vi "Test Cyclic instructions.vi"() -> ()   [LabVIEW 2018]
panel:
  out "Boolean array":bool[](array[boolean])
  out "appended array":string[](array[string])
  in  "String":string="30000"
  in  "cyclic parameter":string
  in  "WPROT positions":cluster{"pos_name":string, "pos_value":dbl}[](array[cluster])=[{"pos_name"="OFFSET", "pos_value"=900.0}, {"pos_name"="WP1", "pos_value"=0.0}, {"pos_name"="WP2", "pos_value"=1875.0}, {"pos_name"="WP3", "pos_value"=3750.0}, {"pos_name"="WP4", "pos_value"=5625.0}, {"pos_name"="WP5", "pos_value"=7500.0}, {"pos_name"="WP6", "pos_value"=9375.0}, {"pos_name"="WP7", "pos_value"=11250.0}, {"pos_name"="WP8", "pos_value"=13125.0}, {"pos_name"="WP9", "pos_value"=15000.0}, {"pos_name"="WP10", "pos_value"=16875.0}, {"pos_name"="WP11", "pos_value"=18750.0}, {"pos_name"="WP12", "pos_value"=20625.0}, {"pos_name"="WP13", "pos_value"=22500.0}, {"pos_name"="WP14", "pos_value"=24375.0}, {"pos_name"="WP15", "pos_value"=26250.0}, {"pos_name"="WP16", "pos_value"=28125.0}] caption="WPROT" {"pos_value" min=-10.0 max=110.0 step=0.1}
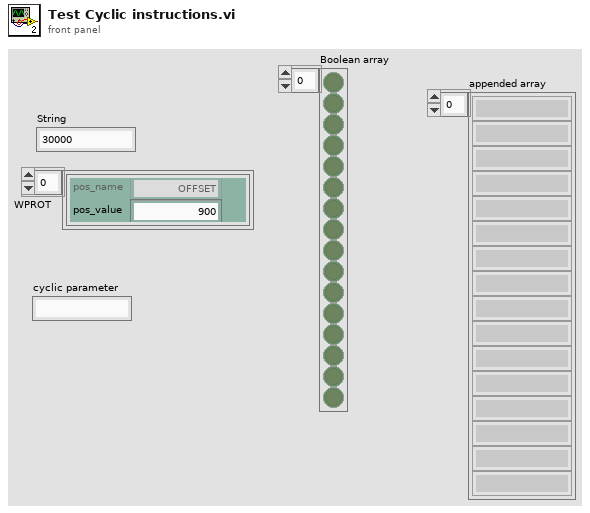
[diagram p1: front panel]
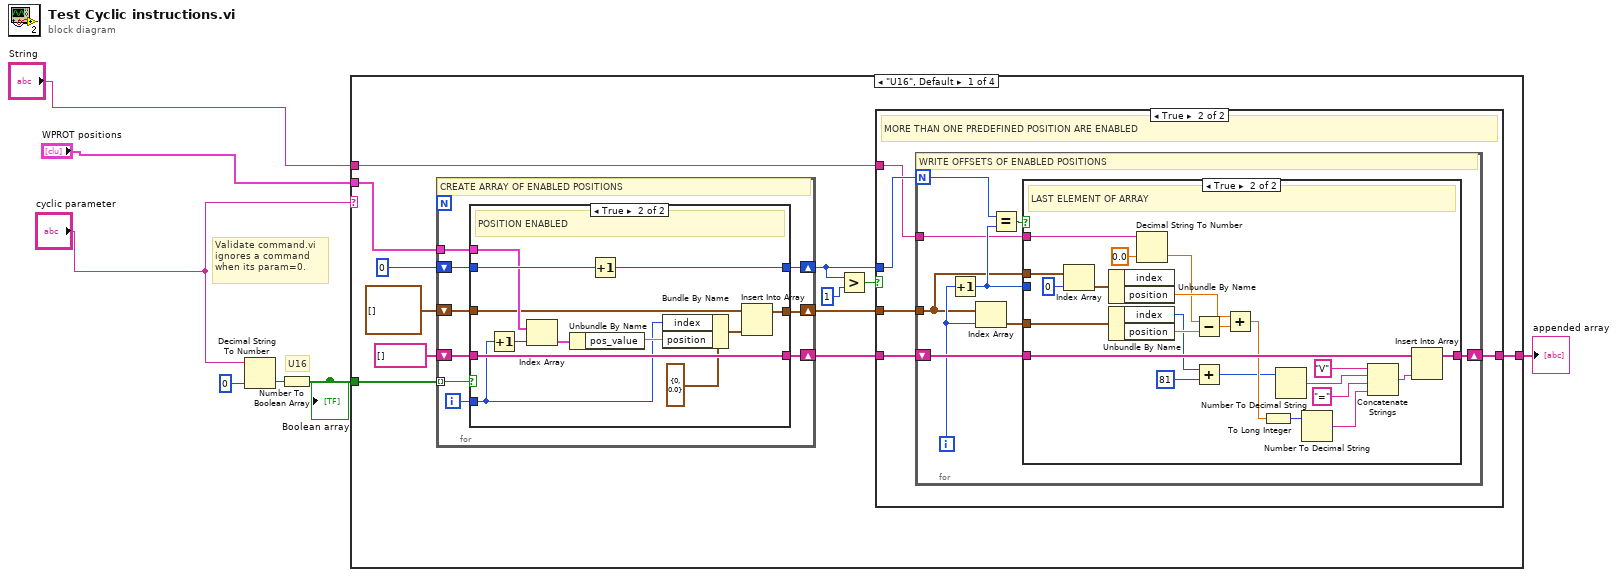
[diagram p0: block diagram]
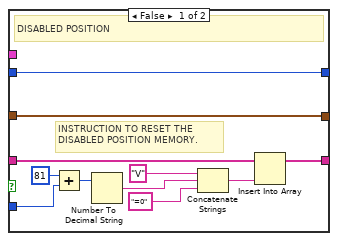
[diagram p2: hidden frame]
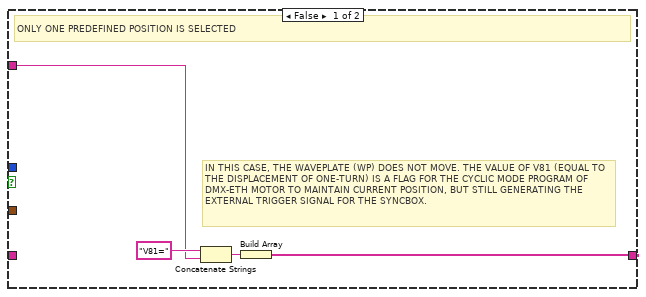
[diagram p3: hidden frame]
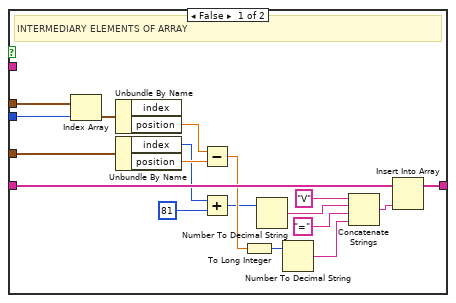
[diagram p4: hidden frame]
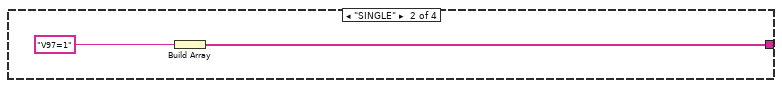
[diagram p5: hidden frame]
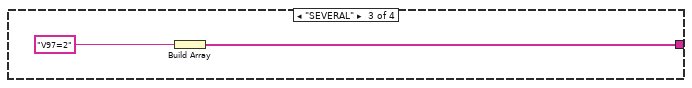
[diagram p6: hidden frame]
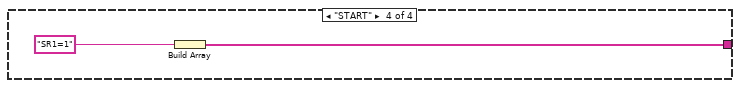
[diagram p7: hidden frame]
diagram:
  # "Validate command.vi\nignores a command\nwhen its param=0."
  # "U16"
  n1 = Decimal String To Number(string="cyclic parameter", default (0L)=u16 0) -> (number=w7:u16)  [unwired: 1 in, 1 out]
  n2 = Number To Boolean Array(number=w7) -> (Boolean array=w5:bool[])
  "Boolean array" <- w5
  n3 = case shown="\"U16\", Default" "cyclic parameter" {
    tunnel: "WPROT positions" -> [w15 _ _ _]
    tunnel: "String" -> [w9 _ _ _]
    tunnel: w5 -> [w17 _ _ _]
    tunnel: [w8 w110 w112 w114] -> w2
    frame "U16", Default {
      n4 = for {
        tunnel: w17 -> [w26] mode=indexing
        shift-right: [w28] -> w10
        shift-left: u16 0 -> [w27]
        shift-right: [w24] -> w11
        shift-left: string[] [] ("appended array") -> [w25]
        tunnel: w15 -> [w22]
        shift-right: [w20] -> w12
        shift-left: cluster{"index":u16, "position":dbl}[] [] ("enabled array") -> [w21]
        i -> [w23]
        # "CREATE ARRAY OF ENABLED POSITIONS"
        n5 = case shown="True" w26 {
          tunnel: [w39 w51] -> w28
          tunnel: w27 -> [w39 w50]
          tunnel: w25 -> [w32 w49]
          tunnel: [w31 w49] -> w24
          tunnel: w23 -> [w33 w40]
          tunnel: w22 -> [_ w48]
          tunnel: w21 -> [w29 w45]
          tunnel: [w29 w46] -> w20
          frame False {
            # "INSTRUCTION TO RESET THE \nDISABLED POSITION MEMORY."
            # "DISABLED POSITION"
            n6 = Add(x=81, y=w33) -> (x+y=w38:i32)
            n7 = Number To Decimal String(number=w38) -> (decimal integer string=w37:string)  [unwired: 1 in]
            n8 = Concatenate Strings("V", w37, "=0") -> (w30:string)
            n9 = Insert Into Array(array=w32, new element=w30) -> (w31:string[])  [unwired: 1 in]
          }
          frame True {
            # "POSITION ENABLED"
            n10 = Increment(x=w40) -> (x+1=w42:i32)
            n11 = Index Array(array=w48, index=w42) -> (element=w47:cluster{"pos_name":string, "pos_value":dbl})
            n12 = Unbundle By Name(w47) -> ("pos_value"=w43:dbl)
            n13 = Increment(x=w50) -> (x+1=w51:u16)
            n14 = Bundle By Name(cluster=cluster{"index":u16, "position":dbl} {"index"=0, "position"=0.0} ("element"), "index"=w40, "position"=w43) -> (w41:cluster{"index":u16, "position":dbl})
            n15 = Insert Into Array(array=w45, new element=w41) -> (w46:cluster{"index":u16, "position":dbl}[])  [unwired: 1 in]
          }
        }
      }
      n16 = Greater?(x=w10, y=u16 1) -> (0:w19:bool)
      n17 = case shown="True" w19 {
        tunnel: w9 -> [w53 w57]
        tunnel: w12 -> [_ w59]
        tunnel: w11 -> [_ w60]
        tunnel: w10 -> [_ w58]
        tunnel: [w52 w56] -> w8
        frame False {
          # "IN THIS CASE, THE WAVEPLATE (WP) DOES NOT MOVE. THE VALUE OF V81 (EQUAL TO THE DISPLACEMENT OF ONE-TURN) IS A FLAG FOR THE CYCLIC MODE PROGRAM OF DMX-ETH MOTOR TO MAINTAIN CURRENT POSITION, BUT STILL GENERATING THE EXTERNAL TRIGGER SIGNAL FOR THE SYNCBOX."
          # "ONLY ONE PREDEFINED POSITION IS SELECTED"
          n18 = Concatenate Strings("V81=", w53) -> (w55:string)
          n19 = Build Array(w55) -> (w52:string[])
        }
        frame True {
          # "MORE THAN ONE PREDEFINED POSITION ARE ENABLED"
          n20 = for {
            N: w58 -> [w65]
            tunnel: w59 -> [w63]
            shift-right: [w66] -> w56
            shift-left: w60 -> [w68]
            tunnel: w57 -> [w61]
            i -> [w67]
            # "WRITE OFFSETS OF ENABLED POSITIONS"
            n21 = Increment(x=w67) -> (x+1=w64:i32)
            n22 = Index Array(array=w63, index=w67) -> (element=w69:cluster{"index":u16, "position":dbl})
            n23 = Equal?(x=w65, y=w64) -> (x = y?=w62:bool)
            n24 = case shown="True" w62 {
              tunnel: w69 -> [w87 w109]
              tunnel: w68 -> [w82 w104]
              tunnel: [w77 w100] -> w66
              tunnel: w64 -> [w75 _]
              tunnel: w63 -> [w74 w99]
              tunnel: w61 -> [_ w89]
              frame False {
                # "INTERMEDIARY ELEMENTS OF ARRAY"
                n25 = Index Array(array=w74, index=w75) -> (element=w73:cluster{"index":u16, "position":dbl})
                n26 = Unbundle By Name(w73) -> ("position"=w76:dbl)  [unwired: 1 out]
                n27 = Unbundle By Name(w87) -> ("index"=w72:u16, "position"=w86:dbl)
                n28 = Subtract(x=w76, y=w86) -> (x-y=w79:dbl)
                n29 = Add(x=w72, y=81 ("x")) -> (x+y=w70:i32)
                n30 = To Long Integer(number=w79) -> (32bit integer=w81:i32)
                n31 = Number To Decimal String(number=w70) -> (decimal integer string=w83:string)  [unwired: 1 in]
                n32 = Number To Decimal String(number=w81) -> (decimal integer string=w80:string)  [unwired: 1 in]
                n33 = Concatenate Strings("V", w83, "=", w80) -> (w78:string)
                n34 = Insert Into Array(array=w82, new element=w78) -> (w77:string[])  [unwired: 1 in]
              }
              frame True {
                # "LAST ELEMENT OF ARRAY"
                n35 = Index Array(array=w99, index=0) -> (element=w98:cluster{"index":u16, "position":dbl})
                n36 = Unbundle By Name(w98) -> ("position"=w95:dbl)  [unwired: 1 out]
                n37 = Unbundle By Name(w109) -> ("index"=w92:u16, "position"=w108:dbl)
                n38 = Decimal String To Number(string=w89, default (0L)=0.0) -> (number=w88:dbl)  [unwired: 1 in, 1 out]
                n39 = Subtract(x=w88, y=w108) -> (x-y=w96:dbl)
                n40 = Add(x=w92, y=u16 81) -> (x+y=w93:u16)
                n41 = Add(x=w95, y=w96) -> (x+y=w94:dbl)
                n42 = To Long Integer(number=w94) -> (32bit integer=w103:i32)
                n43 = Number To Decimal String(number=w93) -> (decimal integer string=w105:string)  [unwired: 1 in]
                n44 = Number To Decimal String(number=w103) -> (decimal integer string=w102:string)  [unwired: 1 in]
                n45 = Concatenate Strings("V", w105, "=", w102) -> (w101:string)
                n46 = Insert Into Array(array=w104, new element=w101) -> (w100:string[])  [unwired: 1 in]
              }
            }
          }
        }
      }
    }
    frame "SINGLE" {
      n47 = Build Array("V97=1" ("string")) -> (w110:string[])
    }
    frame "SEVERAL" {
      n48 = Build Array("V97=2" ("string")) -> (w112:string[])
    }
    frame "START" {
      n49 = Build Array("SR1=1" ("string")) -> (w114:string[])
    }
  }
  "appended array" <- w2
